vi "RandomMCQ_Order(SubVI).vi"(3 "MCQ_Ordered":string[](array[string]), 4 "Question_Ordered":string="1", 5 "connection reference":T1) -> (0 "MCQ_Randomized":string[](array[string]), 2 "connection reference out":T1)   [LabVIEW 2013]
uses:
  <vilib>/addons/database/Connection.llb/Conn ObjectReference.ctl
  <vilib>/addons/database/_DB Variant To Data/Database Variant To Data.xnode
  <vilib>/addons/database/NI_Database_API.lvlib
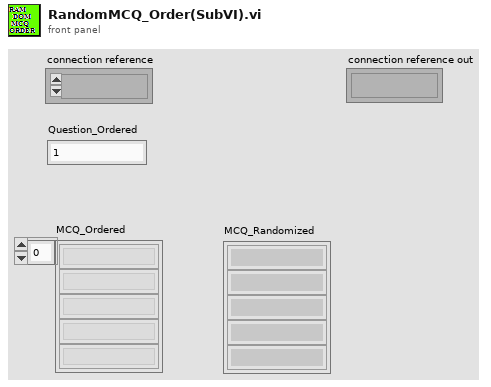
[diagram p1: front panel]
types:
  T1 = typedef "NI_Database_API.lvlib/Conn ObjectReference.ctl" = refnum<k1>
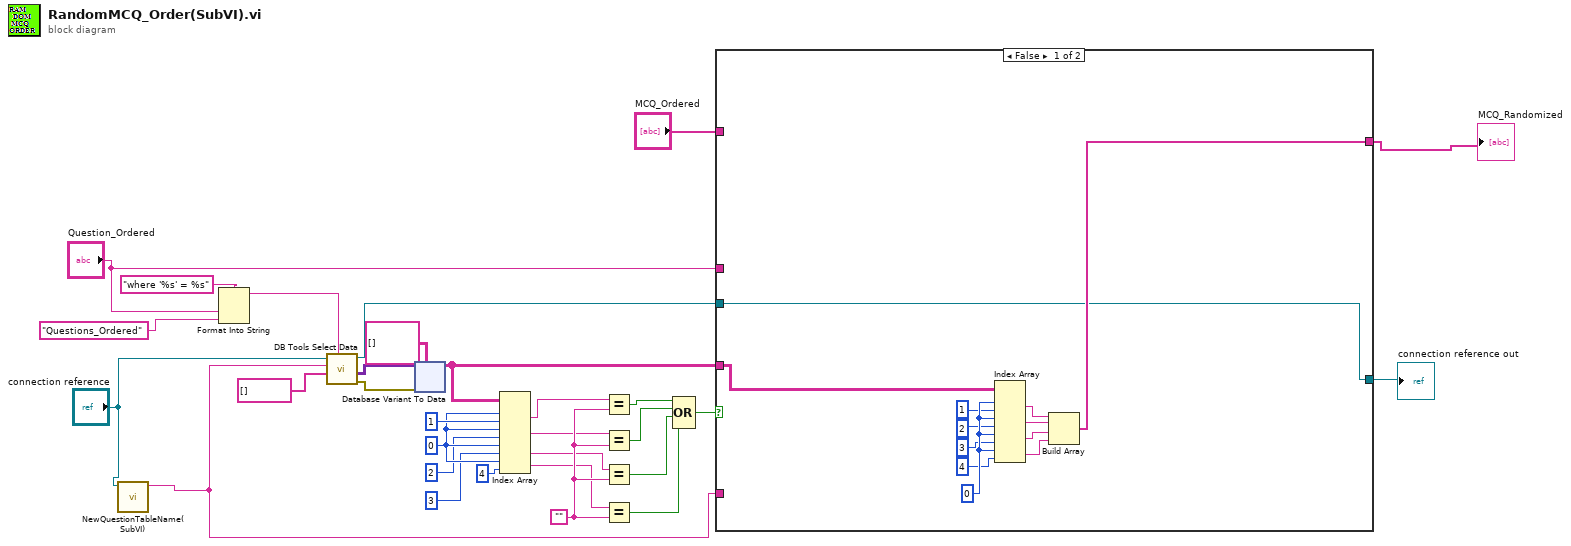
[diagram p0: block diagram]
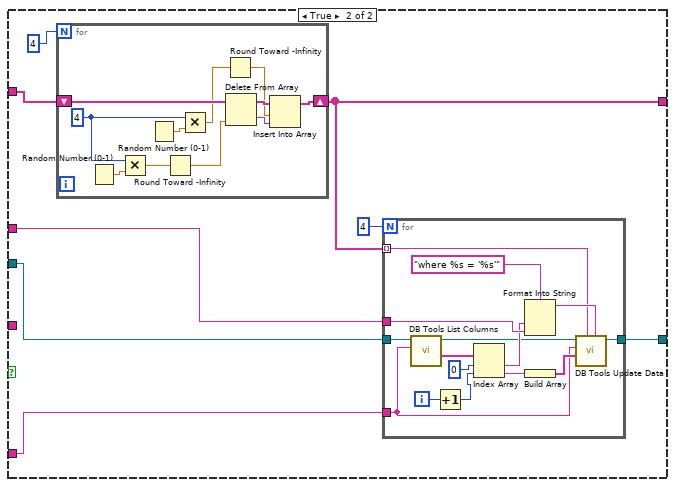
[diagram p2: hidden frame]
diagram:
  w18 = "" ("y")
  w22 = 0 ("index (row)")
  n1 = call "NewQuestionTableName(SubVI).vi"("connection reference"="connection reference") -> ("String"=w2:string)  [unwired: 9 in, 1 out]
  n2 = Format Into String(format string="where '%s' = %s", "Question_Ordered", "Questions_Ordered" ("input 1")) -> (resulting string=w28:string)  [unwired: 2 in, 1 out]
  n3 = call <vilib>:"DB Tools Select Data.vi"("condition"=w28, "columns"=string[] [], "table"=w2, "connection reference"="connection reference") -> ("error out"=w25:errorcluster, "data"=w26:variant[][], "connection reference out"=w7:T1)  [unwired: 2 in]
  n4 = xnode "Database Variant To Data"("database variant"=w26, "error in (no error)"=w25, "type"=string[][] [] ("columns")) -> ("data"=w8:string[][])  [unwired: 1 out]
  n5 = Index Array(array=w8, index (row) #1=w22, index (col) #1=1 ("disabled index (col)"), index (row) #2=w22, index (col) #2=2 ("disabled index (col)"), index (row) #3=w22, index (col) #3=3 ("disabled index (col)"), index (row) #4=w22, index (col) #4=4 ("disabled index (col)")) -> (element #1=w17:string, element #2=w16:string, element #3=w15:string, element #4=w14:string)
  n6 = Equal?(x=w17, y=w18) -> (x = y?=w13:bool)
  n7 = Equal?(x=w16, y=w18) -> (x = y?=w12:bool)
  n8 = Equal?(x=w15, y=w18) -> (x = y?=w11:bool)
  n9 = Equal?(x=w14, y=w18) -> (x = y?=w10:bool)
  n10 = Compound Arithmetic op=OR(w13, w12, w11, w10) -> (w9:bool)
  n11 = case shown="False" w9 {
    tunnel: w2 -> [_ w43]
    tunnel: w8 -> [w33 _]
    tunnel: w7 -> [w31 w44]
    tunnel: "Question_Ordered" -> [_ w45]
    tunnel: "MCQ_Ordered" -> [_ w50]
    tunnel: [w32 w47] -> w3
    tunnel: [w31 w46] -> w4
    frame False {
      w42 = 0 ("index (row)")
      n12 = Index Array(array=w33, index (row) #1=w42, index (col) #1=1, index (row) #2=w42, index (col) #2=2, index (row) #3=w42, index (col) #3=3, index (row) #4=w42, index (col) #4=4) -> (element #1=w37:string, element #2=w36:string, element #3=w35:string, element #4=w34:string)
      n13 = Build Array(w37, w36, w35, w34) -> (w32:string[])
    }
    frame True {
      n14 = for {
        N: 4 ("Numeric") -> [_]
        shift-right: [w72] -> w47
        shift-left: w50 -> [w75]
        w66 = 4
        n15 = Random Number (0-1)() -> (number: 0 to 1=w76:dbl)
        n16 = Multiply(x=w66, y=w76) -> (x*y=w67:dbl)
        n17 = Random Number (0-1)() -> (number: 0 to 1=w71:dbl)
        n18 = Round Toward -Infinity(1:w67) -> (0:w68:dbl)
        n19 = Multiply(x=w66, y=w71) -> (x*y=w69:dbl)
        n20 = Round Toward -Infinity(1:w69) -> (0:w70:dbl)
        n21 = Delete From Array(array=w75, index=w68) -> (deleted portion=w73:string, array with subset deleted=w74:string[])  [unwired: 1 in]
        n22 = Insert Into Array(array=w74, index=w70, new element=w73) -> (w72:string[])
      }
      n23 = for {
        N: 4 -> [_]
        tunnel: w44 -> [w65]
        tunnel: w45 -> [w62]
        tunnel: w47 -> [w52] mode=indexing
        tunnel: [w54] -> w46
        tunnel: w43 -> [w53]
        i -> [w55]
        n24 = call <vilib>:"DB Tools List Columns.vi"("table"=w53, "connection reference"=w65) -> ("columns"=w64:string[], "connection reference out"=w57:T1)  [unwired: 2 in, 2 out]
        n25 = Increment(x=w55) -> (x+1=w51:i32)
        n26 = Index Array(array=w64, index #1=0 ("index"), index #2=w51) -> (element #1=w60:string, element #2=w59:string)
        n27 = Format Into String(format string="where %s = '%s'", w60, w62) -> (resulting string=w56:string)  [unwired: 2 in, 1 out]
        n28 = Build Array(w59) -> (w58:string[])
        n29 = call <vilib>:"DB Tools Update Data.vi"("condition"=w56, "data"=w52, "columns"=w58, "table"=w53, "connection reference"=w57) -> ("connection reference out"=w54:T1)  [unwired: 5 in, 1 out]
      }
    }
  }
  "MCQ_Randomized" <- w3
  "connection reference out" <- w4
